vi "Reset_All_Relay.vi"(8 "error in (no error)":errorcluster caption="entrée d'erreur (pas d'erreur)", 11 "Class Relay_Board usb_relay_device en entrée":refnum<class "Class Relay_Board usb_Relay_device.lvclass">) -> (0 "error out":errorcluster caption="sortie d'erreur", 3 "Class Relay_Board usb_relay_device en sortie":refnum<class "Class Relay_Board usb_Relay_device.lvclass">)   [LabVIEW 2020, in "Library Instrument & Equipement.lvlib" / "Library Relay_Board.lvlib" / "Class Relay_Board usb_Relay_device.lvclass"]
uses:
  Class Relay_Board usb_Relay_device.lvclass
  Class Relay_Board usb_Relay_device.lvclass/Class Relay_Board usb_Relay_device.ctl
  usb_relay_device/usb_relay_device.lvlib
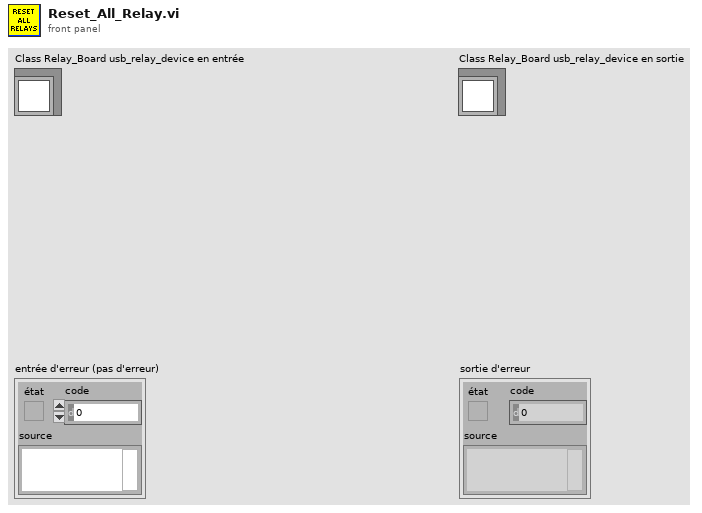
[diagram p1: front panel]
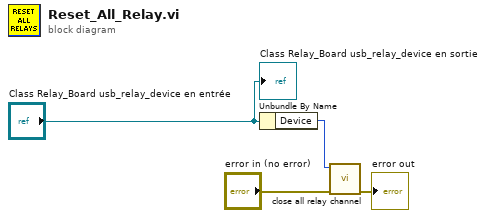
[diagram p0: block diagram]
diagram:
  n1 = Unbundle By Name("Class Relay_Board usb_relay_device en entrée") -> ("Device"=w1:i32)
  n2 = call "close all relay channel.vi"("error in (no error)"="error in (no error)", "hHandle"=w1) -> ("error out"=→"error out":errorcluster)  [unwired: 9 in]
  "Class Relay_Board usb_relay_device en sortie" <- "Class Relay_Board usb_relay_device en entrée"
